vi "EOL CAN_Write Repair Shop Code.vi"(8 "error in":errorcluster, 10 "Read Session in":refnum<k21>, 11 "Write Session in":refnum<k21>) -> (0 "error out":errorcluster, 1 "Rx Message":u8[](array[numeric]), 2 "Response Good?":bool, 3 "TxRxData":string[][](array[string]))   [LabVIEW 2014]
uses:
  Typedefs/Select Session.ctl
  <vilib>/xnet/xnet.llb/XNET Frame CAN.ctl
  <vilib>/xnet/xnet.llb/XNET Frame Type CAN.ctl
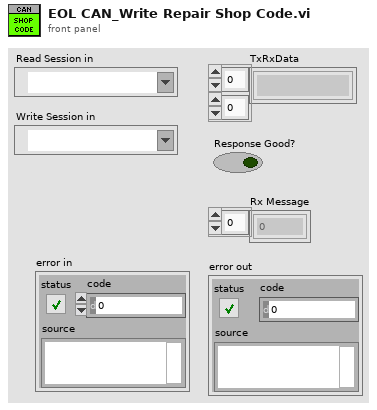
[diagram p1: front panel]
types:
  T1 = typedef "Select Session.ctl" = enum16{"DefaultSession", "Development", "Extended", "EOL", "Programming"}
  T2 = typedef "XNET Frame CAN.ctl" = cluster{"timestamp":timestamp, "payload":u8[], "identifier":u32, "type":T3, "extended?":bool, "echo?":bool}
  T3 = typedef "XNET Frame Type CAN.ctl" = u8
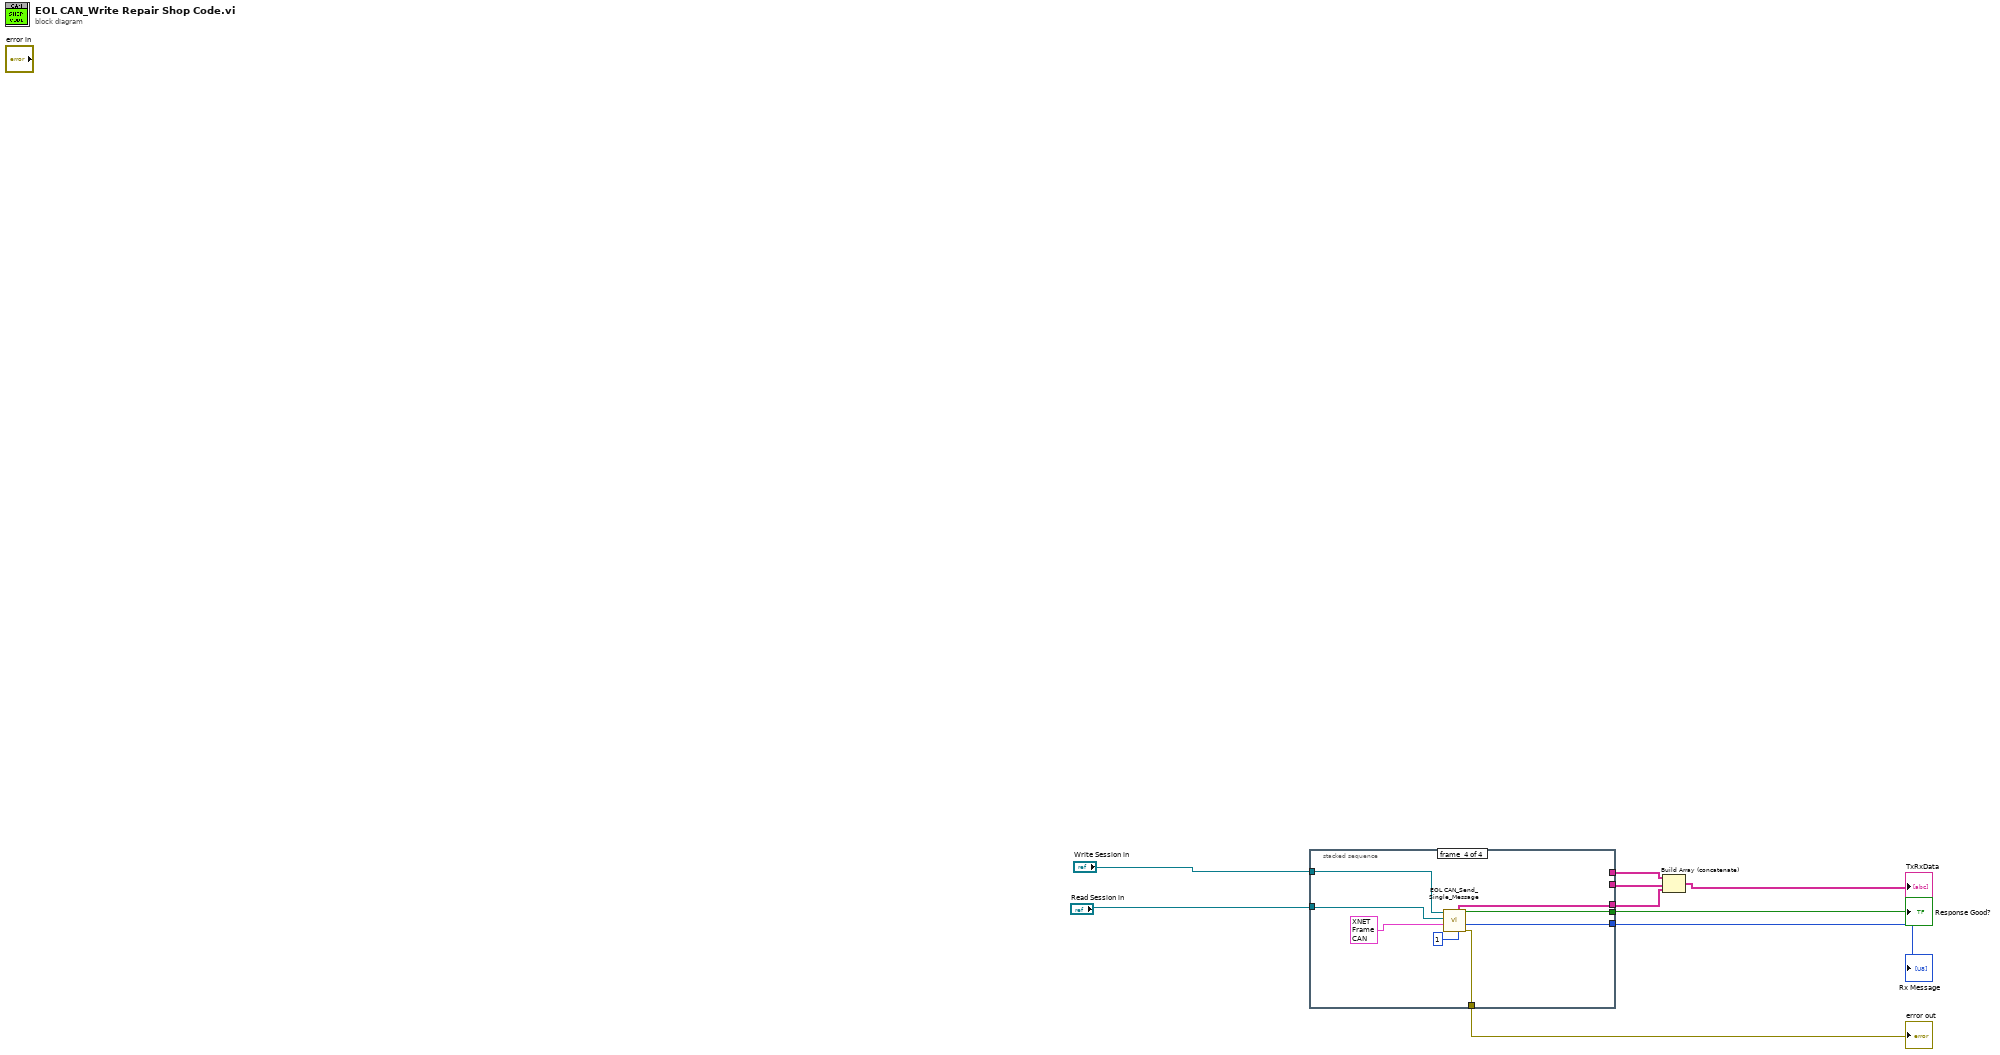
[diagram p0: block diagram]
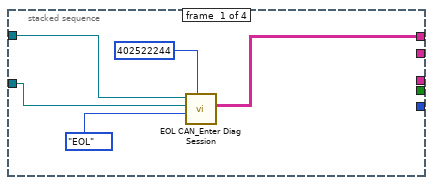
[diagram p2: hidden frame]
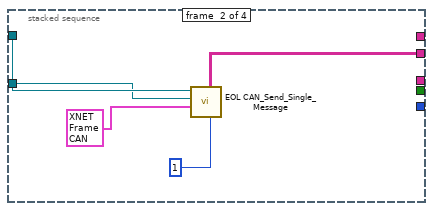
[diagram p3: hidden frame]
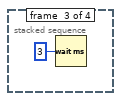
[diagram p4: hidden frame]
diagram:
  n1 = stacked-sequence {
    tunnel: "Write Session in" -> [w12 w19 _ w28]
    tunnel: "Read Session in" -> [w11 w18 _ w27]
    tunnel: [w10 _ _ _] -> w3
    tunnel: [_ w15 _ _] -> w4
    tunnel: [_ _ _ w25] -> w6
    tunnel: [_ _ _ w21] -> w7
    tunnel: [_ _ _ w23] -> w8
    tunnel: [_ _ _ w22] -> w9
    frame #0 {
      n2 = call "EOL CAN_Enter Diag Session.vi"("Rx Arbitration Id"=u32 402522244, "Session"=Select_Session."EOL", "Read Session in"=w11, "Write Session in"=w12) -> ("TxRx Data"=w10:string[][])  [unwired: 5 in, 2 out]
    }
    frame #1 {
      n3 = call "EOL CAN_Send_Single_Message.vi"("Retries"=1, "Tx CAN frame"=T2 {"timestamp"=timestamp(0 s since 1904-01-01), "payload"=[16, 9, 46, 241, 152, 128, 0, 0], "identifier"=402391172, "type"=8, "extended?"=TRUE, "echo?"=FALSE} ("CAN frame"), "Read Session in"=w18, "Write Session in"=w19) -> ("TxRx Data"=w15:string[][])  [unwired: 3 in, 4 out]
    }
    frame #2 {
      n4 = Wait (ms)(milliseconds to wait=u32 3) -> ()  [unwired: 1 out]
    }
    frame #3 {
      n5 = call "EOL CAN_Send_Single_Message.vi"("Retries"=1, "Tx CAN frame"=T2 {"timestamp"=timestamp(0 s since 1904-01-01), "payload"=[33, 0, 29, 101, 85, 85, 85, 85], "identifier"=402391172, "type"=0, "extended?"=TRUE, "echo?"=FALSE} ("CAN frame"), "Read Session in"=w27, "Write Session in"=w28) -> ("Error out"=w25:errorcluster, "Rx Message"=w23:u8[], "Response Good?"=w21:bool, "TxRx Data"=w22:string[][])  [unwired: 3 in, 1 out]
    }
  }
  "Rx Message" <- w8
  "Response Good?" <- w7
  "error out" <- w6
  n6 = Build Array (concatenate)(w3, w4, w9) -> (→"TxRxData":string[][])
